vi "2019-05-09_waveform_2.vi"() -> ()   [LabVIEW 2018]
panel:
  out "웨이브폼 차트 3":T1(graph)={"number: 0 to 1"=0.9752054828416158, "number: 0 to 1"=0.4798579960470657, "number: 0 to 1"=0.8623311878536057}
  out "웨이브폼 차트 2":dbl(graph)=0.4798579960470657
  out "웨이브폼 차트":dbl(graph)=0.9752054828416158
  in  "불리언":bool
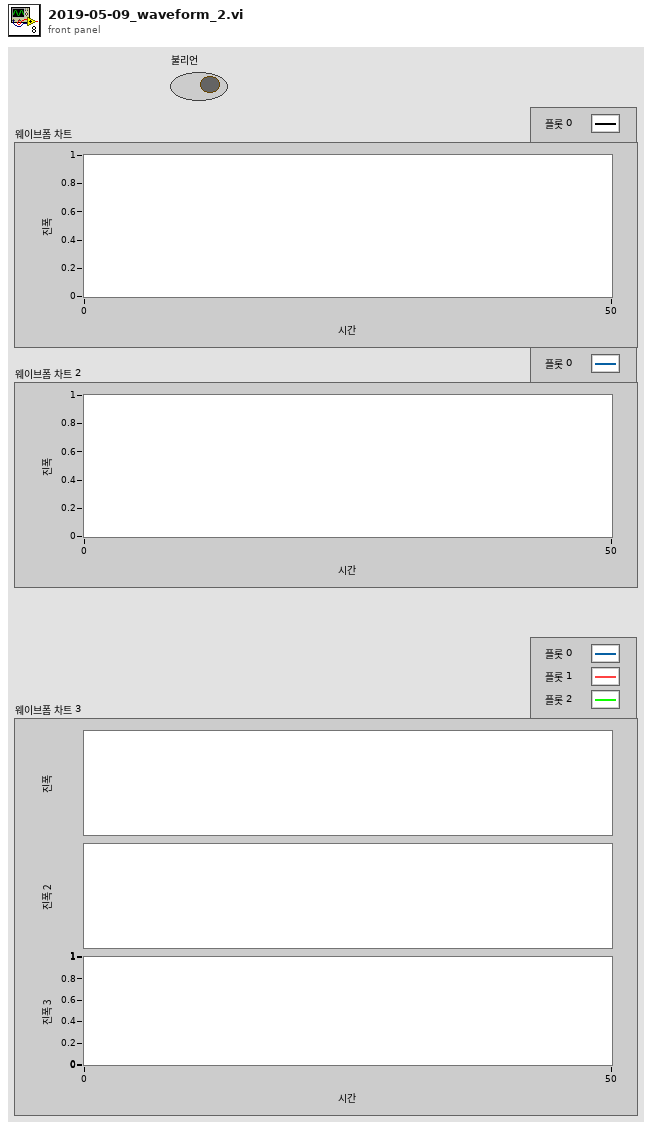
[diagram p1: front panel]
types:
  T1 = cluster{"number: 0 to 1":dbl, "number: 0 to 1":dbl, "number: 0 to 1":dbl}
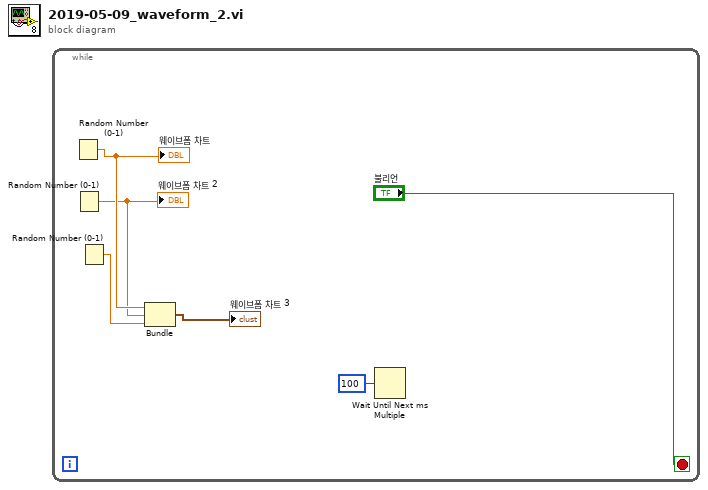
[diagram p0: block diagram]
diagram:
  n1 = while {
    stop <- "불리언" stop-if-true
    n2 = Random Number (0-1)() -> (number: 0 to 1=w5:dbl)
    "웨이브폼 차트" <- w5
    n3 = Random Number (0-1)() -> (number: 0 to 1=w4:dbl)
    "웨이브폼 차트 2" <- w4
    n4 = Random Number (0-1)() -> (number: 0 to 1=w3:dbl)
    n5 = Bundle("number: 0 to 1"=w5, "number: 0 to 1"=w4, "number: 0 to 1"=w3) -> (→"웨이브폼 차트 3":T1)  [unwired: 1 in]
    n6 = Wait Until Next ms Multiple(millisecond multiple=u32 100 ("ms 배수")) -> ()  [unwired: 1 out]
  }
